vi "slopes2zern2diff_test.vi"() -> ()   [LabVIEW 2018]
uses:
  <userlib>/WaveKit.lib/Controls/HasoSlopes.lvclass
panel:
  in  "Hasao slopes file 2":path=path "D:/Data/20200711_AbeComponentCheck/ZernIdx_20_0.has"
  in  "Output folder":path=path "D:/Data/20200711_AbeComponentCheck"
  in  "Output file base name":string="ZernIdx_20_diff"
  in  "Hasao slopes file 1":path=path "D:/Data/20200711_AbeComponentCheck/ZernIdx_20.has"
  out "Zernike pupil":i32[][](graph)
  out "Measured pupil":i32[][](graph)
  out "Diff of Zernike Coefficients":sgl[](graph)
  out "error out":errorcluster
  # "Convert two slopes to Zernike coeffs and calculate the difference: slopes1 - slopes2"
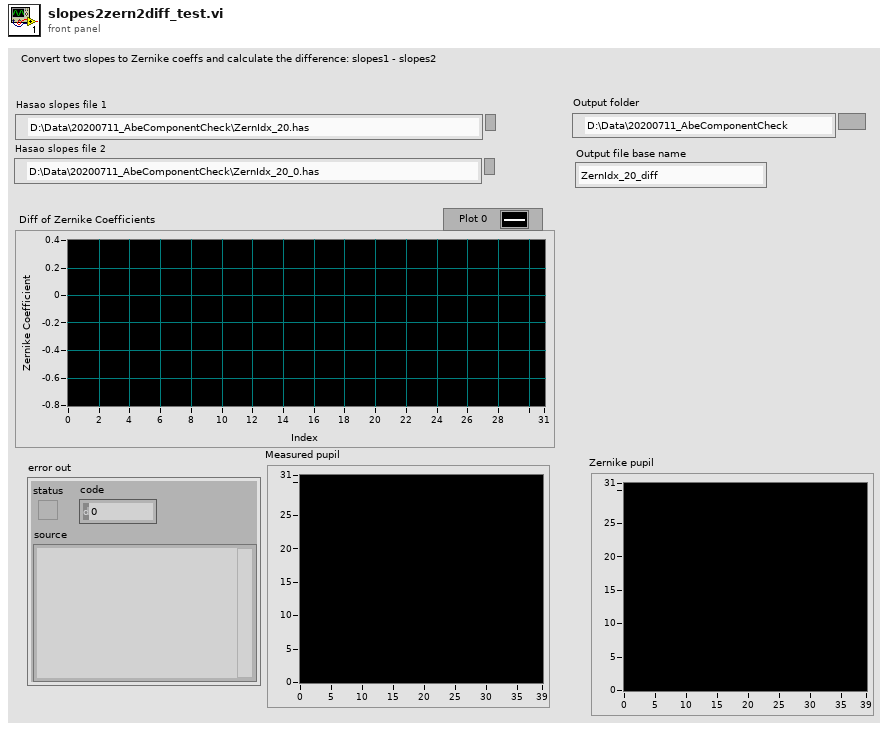
[diagram p1: front panel]
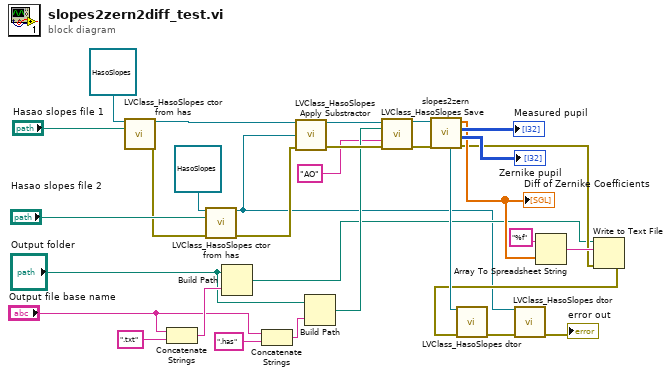
[diagram p0: block diagram]
diagram:
  n1 = call <userlib>:"LVClass_HasoSlopes ctor from has.vi"("HasoSlopes in"=refnum<class "HasoSlopes.lvclass"> refnum, ".has path"="Hasao slopes file 1") -> ("HasoSlopes out"=w11:refnum<class "HasoSlopes.lvclass">, "error out"=w10:errorcluster)  [unwired: 12 in]
  n2 = Concatenate Strings("Output file base name", ".txt") -> (w22:string)
  n3 = call <userlib>:"LVClass_HasoSlopes ctor from has.vi"("HasoSlopes in"=refnum<class "HasoSlopes.lvclass"> refnum, ".has path"="Hasao slopes file 2", "error in (no error)"=w10) -> ("HasoSlopes out"=w1:refnum<class "HasoSlopes.lvclass">, "error out"=w9:errorcluster)  [unwired: 11 in]
  n4 = Build Path(base path="Output folder", name or relative path=w22) -> (appended path=w2:path)
  n5 = Concatenate Strings("Output file base name", ".has") -> (w20:string)
  n6 = call <userlib>:"LVClass_HasoSlopes Apply Substractor.vi"("HasoSlopes in"=w11, "HasoSlopes to substract"=w1, "error in (no error)"=w9) -> ("HasoSlopes out"=w17:refnum<class "HasoSlopes.lvclass">, "error out"=w15:errorcluster)  [unwired: 11 in]
  n7 = Build Path(base path="Output folder", name or relative path=w20) -> (appended path=w14:path)
  n8 = call <userlib>:"LVClass_HasoSlopes Save.vi"("HasoSlopes in"=w17, "path"=w14, "session"="AO", "error in (no error)"=w15) -> ("HasoSlopes out"=w8:refnum<class "HasoSlopes.lvclass">, "error out"=w6:errorcluster)  [unwired: 10 in]
  n9 = call "slopes2zern.vi"("HasoSlopes in"=w8, "error in (no error)"=w6) -> ("HasoSlopes out"=w7:refnum<class "HasoSlopes.lvclass">, "Zernike Coefficients"=w12:sgl[], "Measured pupil"=→"Measured pupil":i32[][], "Zernike pupil"=→"Zernike pupil":i32[][], "error out"=w5:errorcluster)  [unwired: 4 in]
  "Diff of Zernike Coefficients" <- w12
  n10 = Array To Spreadsheet String(array=w12, 3:"%f") -> (spreadsheet string=w28:string)  [unwired: 1 in]
  n11 = Write to Text File(file (use dialog)=w2, text=w28, error in=w5) -> (error out=w4:errorcluster)  [unwired: 1 in, 2 out]
  n12 = call <userlib>:"LVClass_HasoSlopes dtor.vi"("HasoSlopes in"=w7, "error in (no error)"=w4) -> ("error out"=w16:errorcluster)  [unwired: 12 in, 1 out]
  n13 = call <userlib>:"LVClass_HasoSlopes dtor.vi"("HasoSlopes in"=w1, "error in (no error)"=w16) -> ("error out"=→"error out":errorcluster)  [unwired: 12 in, 1 out]
